vi "CameraSerialIDScan.vi"() -> ()   [LabVIEW 2019]
uses:
  <vilib>/vision/driver/NI_Vision_Acquisition_Software.lvlib
panel:
  out "Interface Name":string[](array[string])
  out "Serial Number Low":u32[](array[numeric])
  out "error out":errorcluster
  in  "error in":errorcluster
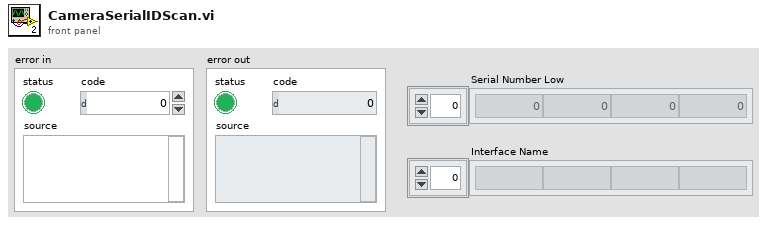
[diagram p1: front panel]
types:
  T1 = cluster{"Type":u32, "Version":u32, "Flags":u32, "SerialNumberHigh":u32, "SerialNumberLow":u32, "BusType":u32, "InterfaceName":string, "VendorName":string, "ModelName":string, "CameraFileName":string, "CameraAttributeURL":string}[]
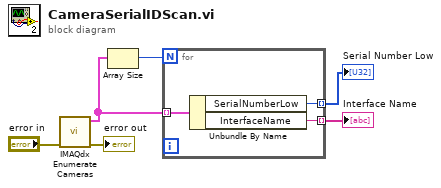
[diagram p0: block diagram]
diagram:
  n1 = call <vilib>:"IMAQdx Enumerate Cameras.vi"("error in"="error in") -> ("error out"=→"error out":errorcluster, "Camera Information Array"=w5:T1)  [unwired: 9 in]
  n2 = Array Size(array=w5) -> (size(s)=w6:i32)
  n3 = for {
    N: w6 -> [_]
    tunnel: w5 -> [w9] mode=indexing
    tunnel: [w8] -> w2 mode=indexing
    tunnel: [w7] -> w1 mode=indexing
    n4 = Unbundle By Name(w9) -> ("SerialNumberLow"=w8:u32, "InterfaceName"=w7:string)
  }
  "Serial Number Low" <- w2
  "Interface Name" <- w1
